vi "004 Recta.vi"() -> ()   [LabVIEW 2019]
panel:
  in  "stop":bool
  out "n":dbl format="%#_4g"
  out "m":dbl format="%#_4g"
  in  "Y2":dbl
  in  "X2":dbl
  in  "Y1":dbl
  in  "X1":dbl
  # "RECTA:\nCalcula una recta a partir de dos punts: (X1, Y1) (X2, Y2)"
  # "· x  +"
  # "y ="
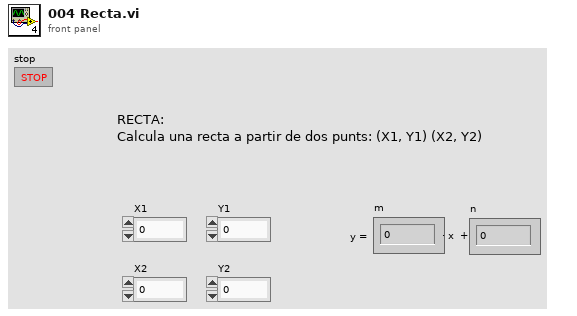
[diagram p1: front panel]
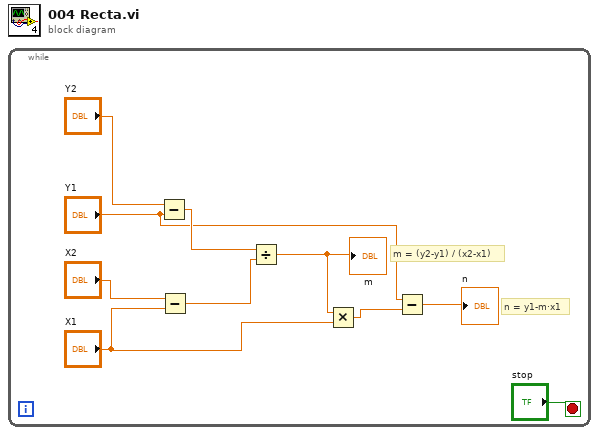
[diagram p0: block diagram]
diagram:
  n1 = while {
    stop <- "stop" stop-if-true
    # "m = (y2-y1) / (x2-x1)"
    # "n = y1-m·x1"
    n2 = Subtract(x="Y2", y="Y1") -> (x-y=w8:dbl)
    n3 = Subtract(x="X2", y="X1") -> (x-y=w7:dbl)
    n4 = Divide(x=w8, y=w7) -> (x/y=w6:dbl)
    "m" <- w6
    n5 = Multiply(x=w6, y="X1") -> (x*y=w4:dbl)
    n6 = Subtract(x="Y1", y=w4) -> (x-y=→"n":dbl)
  }
